vi "DrawTopics.vi"(5 "Registered":T1[](array[typedef]), 6 "Status":T3[](array[typedef]), 7 "Selection":i32) -> (0 "new picture":picture, 1 "Status":string, 2 "all good?":bool, 3 "Boundaries":cluster{i32, i32}[](array[cluster])=[{10, 22}, {30, 42}, {50, 62}], 4 "Key":picture)   [LabVIEW 2014]
doc: "Record state of running topics to the Master console"
uses:
  <userlib>/ROS for LabVIEW Software/ROS/Code/Console/Servers/ServerSubs/MyState.ctl
  <userlib>/ROS for LabVIEW Software/ROS/Code/SubVIs/_ROSControl.ctl
  <userlib>/ROS for LabVIEW Software/ROS/Code/SubVIs/_ROSDirection.ctl
  <vilib>/Utility/miscctls.llb/LVRectTypeDef.ctl
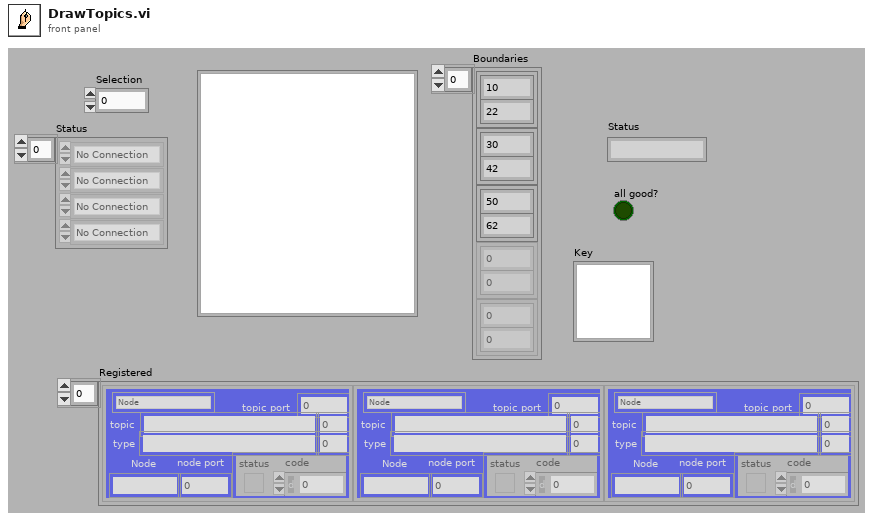
[diagram p1: front panel]
types:
  T1 = typedef "_ROSControl.ctl" = cluster{"topic port":u16, "Node":string, "topic":string, "type":string, "node port":u16, "error ":errorcluster, "Direction":T2, "Update (ms)":u16, "FIFO size":u16}
  T2 = typedef "_ROSDirection.ctl" = enum16{"Node", "Publisher", "Subscriber", "ServiceClient", "ServiceProvider"}
  T3 = typedef "MyState.ctl" = enum16{"No Connection", "Registered", "Connected", "Close"}
  T4 = cluster{"left":i16, "top":i16, "right":i16, "bottom":i16}
  T5 = typedef "LVRectTypeDef.ctl" = cluster{"Left":i16, "Top":i16, "Right":i16, "Bottom":i16}
  T6 = typedef "imagedata.ctl" = cluster{"image type":i32, "image depth":i32, "image":u8[], "mask":u8[], "colors":u32[], "Rectangle":cluster{"left":i16, "top":i16, "right":i16, "bottom":i16}}
  T7 = cluster{"horizontal":enum16{"left", "center", "right"}, "vertical":enum16{"top", "center", "bottom"}}
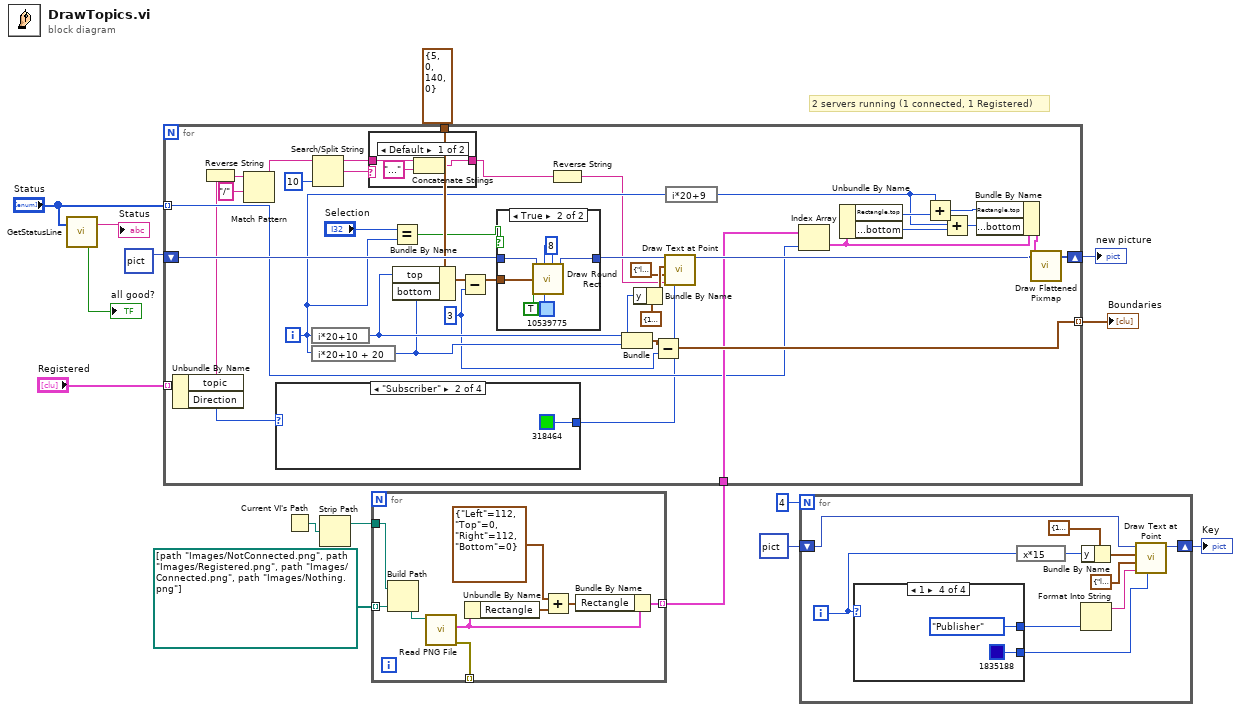
[diagram p0: block diagram]
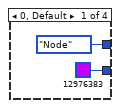
[diagram p2: hidden frame]
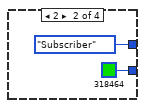
[diagram p3: hidden frame]
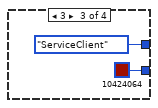
[diagram p4: hidden frame]
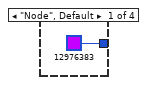
[diagram p5: hidden frame]
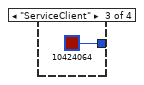
[diagram p6: hidden frame]
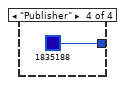
[diagram p7: hidden frame]
diagram:
  # "2 servers running (1 connected, 1 Registered)"
  n1 = call <userlib>:"GetStatusLine.vi"("Status"="Status") -> ("all good?"=→"all good?":bool, "Status"=→"Status":string)  [unwired: 1 in]
  n2 = Current VI's Path() -> (path=w10:path)
  n3 = Strip Path(path=w10) -> (stripped path=w9:path)  [unwired: 1 out]
  n4 = for {
    tunnel: [w22] -> w11 mode=indexing
    tunnel: w9 -> [w19]
    tunnel: path[] [path "Images/NotConnected.png", path "Images/Registered.png", path "Images/Connected.png", path "Images/Nothing.png"] -> [w18] mode=indexing
    tunnel: [w16] -> _ mode=indexing
    n5 = Build Path(base path=w19, name or relative path=w18) -> (appended path=w17:path)
    n6 = call <vilib>:"Read PNG File.vi"("path to PNG file"=w17) -> ("error out"=w16:errorcluster, "image data"=w23:T6)  [unwired: 8 in, 1 out]
    n7 = Unbundle By Name(w23) -> ("Rectangle"=w21:T4)
    n8 = Add(x=T5 {"Left"=112, "Top"=0, "Right"=112, "Bottom"=0} ("Bounds"), y=w21) -> (x+y=w20:T5)
    n9 = Bundle By Name(cluster=w23, "Rectangle"=w20) -> (w22:T6)
  }
  n10 = for {
    shift-right: [w48] -> w15
    shift-left: picture data[5B] ("new picture") -> [w59]
    tunnel: [w54] -> w13 mode=indexing
    tunnel: T4 {"left"=5, "top"=0, "right"=140, "bottom"=0} ("rect") -> [w55]
    tunnel: w11 -> [w46]
    tunnel: "Status" -> [w37] mode=indexing
    tunnel: "Registered" -> [w28] mode=indexing
    i -> [w41]
    w51 = i16 3 ("oval width")
    n11 = Unbundle By Name(w28) -> ("topic"=w27:string, "Direction"=w26:T2)
    n12 = Reverse String(1:w27) -> (0:w36:string)
    n13 = Match Pattern(string=w36, regular expression="/") -> (before substring=w33:string)  [unwired: 1 in, 3 out]
    n14 = case shown="\"Subscriber\"" w26 {
      tunnel: [u32 12976383 ("color(black)") u32 318464 ("color(black)") u32 10424064 ("color(black)") u32 1835188 ("color(black)")] -> w25
      frame "Node", Default {
      }
      frame "Subscriber" {
      }
      frame "ServiceClient" {
      }
      frame "Publisher" {
      }
    }
    n15 = expression code="i*20+10"(w41) -> (w57:i32)
    n16 = expression code="i*20+10 + 20"(w41) -> (w56:i32)
    n17 = Search/Split String(string=w33, offset (0)=10) -> (substring before match=w29:string, match + rest of string=w31:string)  [unwired: 1 in, 1 out]
    n18 = case shown="Default" w31 {
      tunnel: [w70 w71] -> w30
      tunnel: w29 -> [w69 w71]
      frame Default {
        n19 = Concatenate Strings(w69, "..." ("string")) -> (w70:string)
      }
      frame "" {
      }
    }
    n20 = Equal?(x="Selection", y=w41) -> (x = y?=w49:bool)
    n21 = Bundle By Name(cluster=w55, "top"=w57, "bottom"=w56) -> (w53:T4)
    n22 = Subtract(x=w53, y=w51) -> (x-y=w52:T4)
    n23 = case shown="True" w49 {
      tunnel: w59 -> [w72 w75]
      tunnel: [w72 w74] -> w58
      tunnel: w52 -> [_ w73]
      frame False {
      }
      frame True {
        w76 = i16 8 ("oval width")
        n24 = call <vilib>:"Draw Round Rect.vi"("picture"=w75, "oval width"=w76, "rect"=w73, "fill?(F)"=TRUE, "color(black)"=u32 10539775, "oval height"=w76) -> ("new picture"=w74:picture)  [unwired: 3 in]
      }
    }
    n25 = Reverse String(1:w30) -> (0:w34:string)
    n26 = Bundle(w57, w56) -> (w61:cluster{i32, i32})  [unwired: 1 in]
    n27 = Bundle By Name(cluster=cluster{"x":i16, "y":i16} {"x"=10, "y"=0} ("origin"), "y"=w57) -> (w62:cluster{"x":i16, "y":i16})
    n28 = Subtract(x=w61, y=w51) -> (x-y=w54:cluster{i32, i32})
    n29 = call <vilib>:"Draw Text at Point.vi"("text color(black)"=w25, "text"=w34, "alignment(left, top)"=T7 {"horizontal"=enum."left", "vertical"=enum."top"}, "origin"=w62, "picture"=w58) -> ("new picture"=w47:picture)  [unwired: 5 in, 1 out]
    n30 = expression code="i*20+9"(w41) -> (w39:i32)
    n31 = Index Array(array=w46, index=w37) -> (element=w42:T6)
    n32 = Unbundle By Name(w42) -> ("Rectangle.top"=w44:i16, "Rectangle.bottom"=w40:i16)
    n33 = Add(x=w39, y=w44) -> (x+y=w45:i32)
    n34 = Add(x=w40, y=w39) -> (x+y=w38:i32)
    n35 = Bundle By Name(cluster=w42, "Rectangle.top"=w45, "Rectangle.bottom"=w38) -> (w43:T6)
    n36 = call <vilib>:"Draw Flattened Pixmap.vi"("image data"=w43, "picture"=w47) -> ("new picture"=w48:picture)  [unwired: 7 in]
  }
  "new picture" <- w15
  "Boundaries" <- w13
  n37 = for {
    N: 4 -> [_]
    shift-right: [w82] -> w1
    shift-left: picture data[5B] ("new picture") -> [w81]
    i -> [w84]
    n38 = case shown="1" w84 {
      tunnel: [u32 12976383 ("color(black)") u32 318464 ("color(black)") u32 10424064 ("color(black)") u32 1835188 ("color(black)")] -> w80
      tunnel: [_ROSDirection."Node" ("Direction") _ROSDirection."Subscriber" ("Direction") _ROSDirection."ServiceClient" ("Direction") _ROSDirection."Publisher" ("Direction")] -> w79
      frame 0, Default {
      }
      frame 2 {
      }
      frame 3 {
      }
      frame 1 {
      }
    }
    n39 = expression code="x*15"(w84) -> (w83:i32)
    n40 = Format Into String(w79) -> (resulting string=w85:string)  [unwired: 3 in, 1 out]
    n41 = Bundle By Name(cluster=cluster{"x":i16, "y":i16} {"x"=10, "y"=0} ("origin"), "y"=w83) -> (w87:cluster{"x":i16, "y":i16})
    n42 = call <vilib>:"Draw Text at Point.vi"("text color(black)"=w80, "text"=w85, "alignment(left, top)"=T7 {"horizontal"=enum."left", "vertical"=enum."top"}, "origin"=w87, "picture"=w81) -> ("new picture"=w82:picture)  [unwired: 5 in, 1 out]
  }
  "Key" <- w1
